vi "Get Item Property (Dependent File).vi"(8 "error in (no error)":errorcluster, 10 "Property Name":string, 11 "Item Ref in":T2 format="%.0x") -> (0 "error out":errorcluster, 1 "Path":path, 3 "Item Ref out":T2 format="%.0x", 4 "Found":bool, 5 "OptionalInfo":T1)   [LabVIEW 2020, in "Custom Device API.lvlib"]
doc: "Returns the <B>Value</B> of a specific item <B>Property Name</B>. Properties do not inherit within a custom device, so <B>Item Ref in</B> must reference the specific item on which the property is set. \n\nFor instances with a <B>Default Value</B> input, the <B>Value</B> output returns this value if the <B>Property Name</B> is not found for the specified item. Wire data to the <B>Default Value</B> input to determine the polymorphic instance to use or manually select the instance."
uses:
  <vilib>/NI VeriStand/Custom Device API/Custom Device API.lvlib
  <vilib>/NI VeriStand/Custom Device API/Custom Device Item Ref.ctl
  <vilib>/NI VeriStand/Custom Device API/Dependent File Optional Info.ctl
  417ec2ff-9618-4f9d-89b2-1b865676f7d1.vi
  <vilib>/NI VeriStand/Custom Device API/Custom Device Offline Path.vi
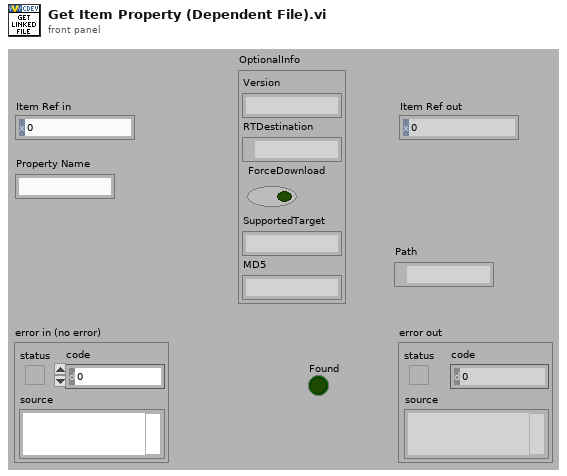
[diagram p1: front panel]
types:
  T1 = typedef "Custom Device API.lvlib/Dependent File Optional Info.ctl" = cluster{"Version":string, "RTDestination":path, "ForceDownload":bool, "SupportedTarget":string, "MD5":string}
  T2 = typedef "Custom Device API.lvlib/Custom Device Item Ref.ctl" = u64
  T3 = typedef "Tree Storage.lvlib/OptionalDependentFileType.ctl" = cluster{"Version":string, "RTDestination":path, "ForceDownload":bool, "SupportedTarget":string, "MD5":string}
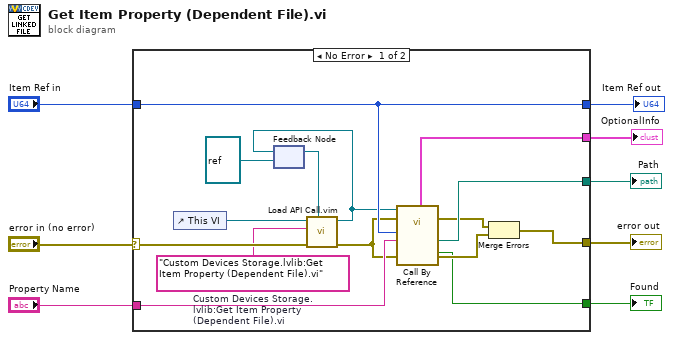
[diagram p0: block diagram]
diagram:
  n1 = case shown="No Error" "error in (no error)" {
    selector: "error in (no error)" -> [w14 w24]
    tunnel: "Item Ref in" -> [w17 w25]
    tunnel: [w17 w25] -> w7
    tunnel: [w22 w24] -> w6
    tunnel: "Property Name" -> [w21 _]
    tunnel: [w20 _] -> w4
    tunnel: [w19 _] -> w3
    tunnel: [w18 _] -> w2
    frame No Error {
      w11 = "Custom Devices Storage.lvlib:Get Item Property (Dependent File).vi"  # Custom Devices Storage.lvlib:Get Item Property (Dependent File).vi
      n2 = control-ref of="This VI"() -> (w15:refnum<vi>)
      n3 = feedback #1(refnum<vi> refnum ("type specifier VI Refnum (for type only)")) -> (w16:refnum<vi>)
      n4 = call "Load API Call.vim"("VI reference in"=w16, "error in (no error)"=w14, "VI qualified name"=w11, "Caller VI ref"=w15) -> ("error out"=w13:errorcluster, "VI reference"=w12:refnum<vi>)  [unwired: 6 in]
      n5 = feedback-in #1(w12) -> ()
      n6 = call-by-ref "?"(reference=w12, error in=w13, 8:"error in (no error)"=w13, "Property Name"=w21, "Item Ref in"=w17) -> (error out=w9:errorcluster, 0:"error out"=w23:errorcluster, "Path"=w19:path, "Found?"=w20:bool, "OptionalInfo"=w18:T3)  [unwired: 4 in, 2 out]
      n7 = Merge Errors(w9, w23) -> (w22:errorcluster)
    }
    frame Error {
    }
  }
  "Item Ref out" <- w7
  "error out" <- w6
  "Path" <- w3
  "Found" <- w4
  "OptionalInfo" <- w2
